vi "SetControlVisibilityAndEnabledState.vi"(6 "error in (no error)":errorcluster, 8 "Enabled state (Enabled)":T2(ring), 9 "Visible (T)":bool=TRUE, 10 "Ctl Refnum":refnum<vi>, 11 "Control State Array":T1[](array[typedef])) -> (0 "error out":errorcluster, 3 "Control State Array (out)":T1[](array[typedef]))   [LabVIEW 2017]
doc: "Modifies state variable of the control indicated by the reference. States are: Visible (T/F), Enabled (Enabled, Disabled, Disabled and greyed out)"
uses:
  Types/ControlAttributes.ctl
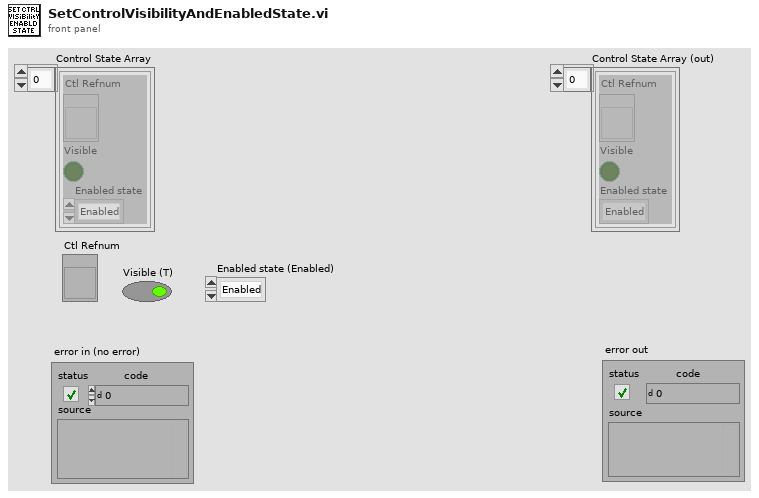
[diagram p1: front panel]
types:
  T1 = typedef "ControlAttributes.ctl" = cluster{"Ctl Refnum":refnum<vi>, "Visible":bool, "Enabled state":enum8{"Enabled", "Disabled", "Disabled and Grayed Out"}}
  T2 = enum8{"Enabled", "Disabled", "Disabled and Grayed Out"}
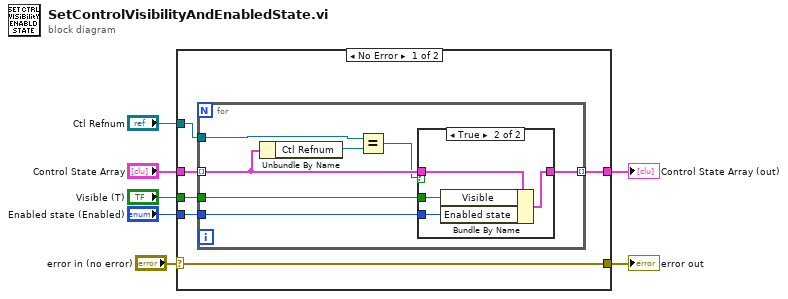
[diagram p0: block diagram]
diagram:
  n1 = case shown="No Error" "error in (no error)" {
    selector: "error in (no error)" -> [w13 w27]
    tunnel: [w13 w27] -> w6
    tunnel: "Control State Array" -> [w12 w26]
    tunnel: "Ctl Refnum" -> [w11 _]
    tunnel: "Enabled state (Enabled)" -> [w10 _]
    tunnel: "Visible (T)" -> [w9 _]
    tunnel: [w8 w26] -> w1
    frame No Error {
      n2 = for {
        tunnel: w12 -> [w18] mode=indexing
        tunnel: w11 -> [w19]
        tunnel: w10 -> [w15]
        tunnel: w9 -> [w16]
        tunnel: [w17] -> w8 mode=indexing
        n3 = Unbundle By Name(w18) -> ("Ctl Refnum"=w20:refnum<vi>)
        n4 = Equal?(x=w19, y=w20) -> (x = y?=w14:bool)
        n5 = case shown="True" w14 {
          tunnel: w18 -> [w21 w25]
          tunnel: [w21 w24] -> w17
          tunnel: w16 -> [_ w23]
          tunnel: w15 -> [_ w22]
          frame False {
          }
          frame True {
            n6 = Bundle By Name(cluster=w25, "Visible"=w23, "Enabled state"=w22) -> (w24:T1)
          }
        }
      }
    }
    frame Error {
    }
  }
  "error out" <- w6
  "Control State Array (out)" <- w1
